vi "Serve Buffer.vi"(7 "transfer id":i32, 8 "error in (no error)":errorcluster, 9 "group id":i32, 10 "plugin id":i32, 11 "Data Server Thread in":refnum<class "Data Server Thread.lvclass">) -> (0 "error out":errorcluster, 3 "Data Server Thread out":refnum<class "Data Server Thread.lvclass">)   [LabVIEW 2017, in "DSF Core.lvlib" / "Data Server Thread.lvclass"]
uses:
  Data Server Thread.lvclass
  Data Server Thread.lvclass/Data Server Thread.ctl
  Buffer Map/Buffers Map.lvclass
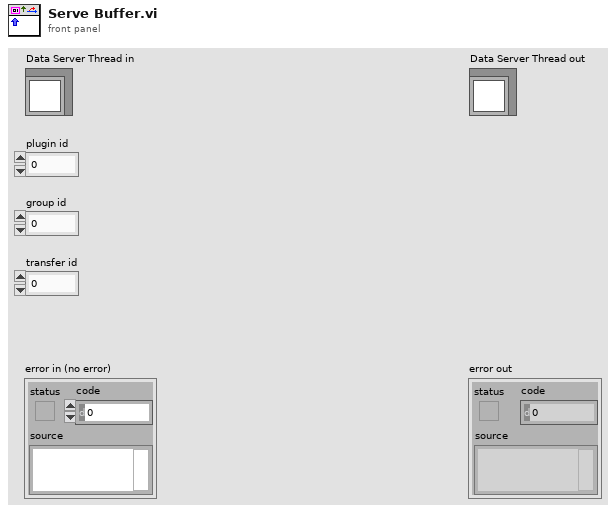
[diagram p1: front panel]
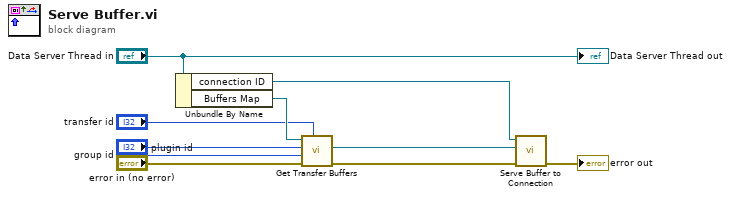
[diagram p0: block diagram]
diagram:
  n1 = Unbundle By Name("Data Server Thread in") -> ("connection ID"=w2:refnum<k5>, "Buffers Map"=w6:refnum<class "Buffers Map.lvclass">)
  n2 = call "Get Transfer Buffers.vi"("transfer id"="transfer id", "error in (no error)"="error in (no error)", "group id"="group id", "plugin id"="plugin id", "Buffers Map in"=w6) -> ("error out"=w4:errorcluster, "engine Buffer"=w1:refnum<class "Buffer.lvclass">)  [unwired: 3 in, 2 out]
  n3 = call "Serve Buffer to Connection.vi"("error in (no error)"=w4, "Buffer"=w1, "connection ID in"=w2) -> ("error out"=→"error out":errorcluster)  [unwired: 7 in, 1 out]
  "Data Server Thread out" <- "Data Server Thread in"
